vi "Replace.vi"(6 "Variant in":variant caption="变体输入", 7 "Shift Pressed?":bool caption="按下Shift？", 8 "error in (no error)":errorcluster caption="错误输入（无错误）", 10 "QD Combo Box Ref":refnum<vi> caption="快速放置组合框引用", 11 "QD Launch VI Ref":refnum<vi> caption="快速放置启动VI引用") -> (0 "error out":errorcluster caption="错误输出", 4 "Variant out":variant caption="变体输出")   [LabVIEW 2016]
doc: "将前面板或程序框图中选定的对象替换为快速放置对话框中通过名称指定的对象。\n\n默认快捷键 - [P]"
panel:
  in  "Select a Control":string="选择控件..." caption="选择控件"
  in  "Select a VI":string="选择VI..." caption="选择VI"
  in  "Undo Name":string="替换" caption="撤消名称"
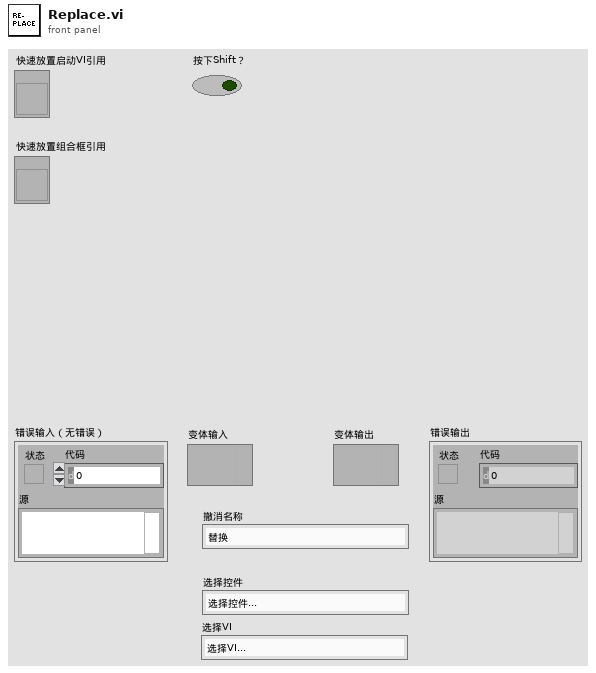
[diagram p1: front panel]
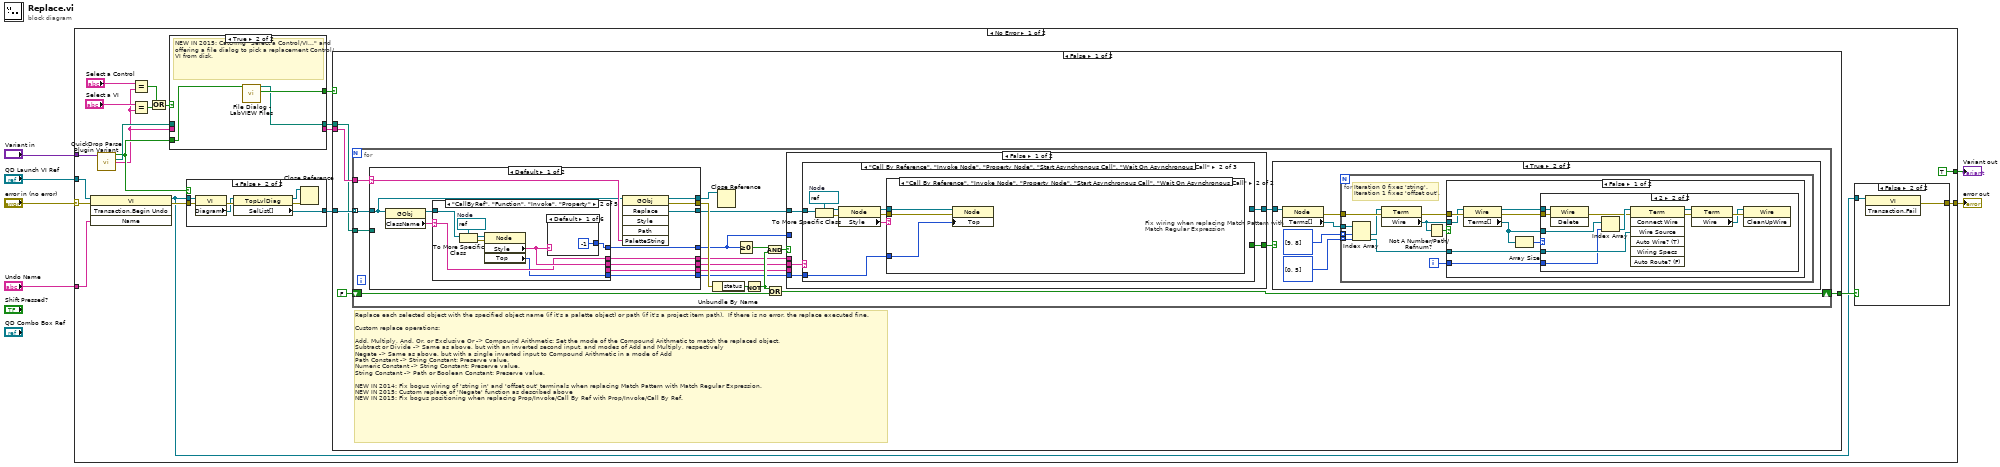
[diagram p0: block diagram]
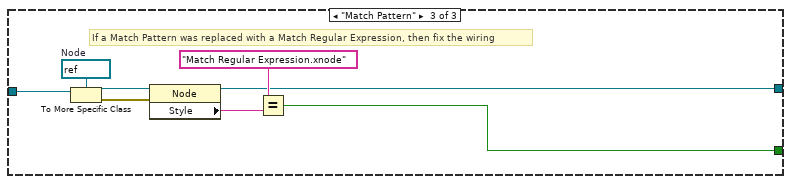
[diagram p7: hidden frame]
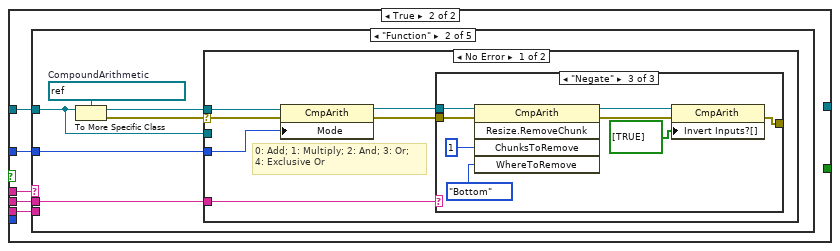
[diagram p8: hidden frame]
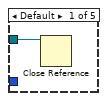
[diagram p9: hidden frame]
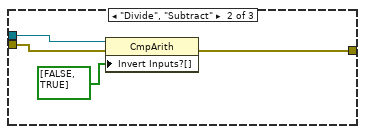
[diagram p11: hidden frame]
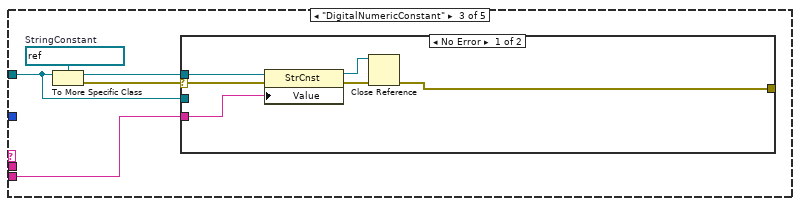
[diagram p13: hidden frame]
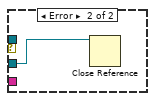
[diagram p14: hidden frame]
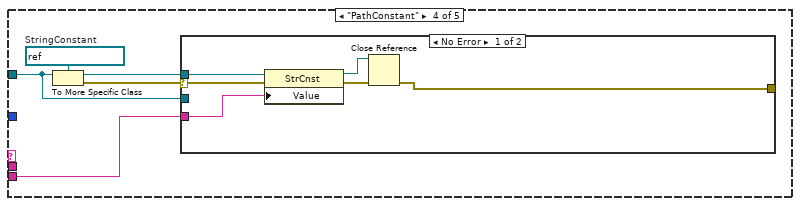
[diagram p15: hidden frame]
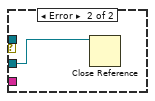
[diagram p16: hidden frame]
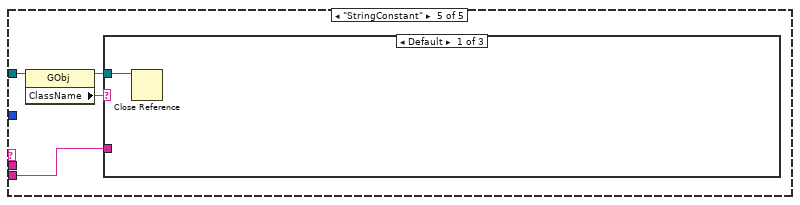
[diagram p17: hidden frame]
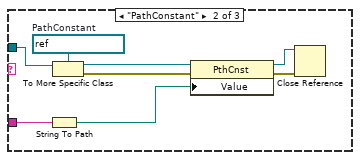
[diagram p18: hidden frame]
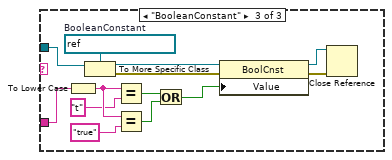
[diagram p19: hidden frame]
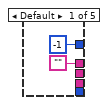
[diagram p20: hidden frame]
diagram:
  n1 = case shown="No Error" "error in (no error)" {
    selector: "error in (no error)" -> [w26 w271]
    tunnel: [w21 w271] -> w5
    tunnel: "QD Launch VI Ref" -> [w25 _]
    tunnel: "Variant in" -> [w27 _]
    tunnel: "Undo Name" -> [w24 _]
    tunnel: [TRUE _] -> w1
    frame No Error {
      n2 = invoke class="VI" method="Transaction.Begin Undo"(reference=w25, error in=w26, "Name"=w24) -> (reference out=w13:refnum<vi>, error out=w22:errorcluster)  [unwired: 1 in, 2 out]
      n3 = call <vilib>:"QuickDrop Parse Plugin Variant.vi"("QDKS Variant in"=w27) -> ("QD Launch VI Panel?"=w11:bool, "Project VI Path"=w15:path, "Palette Object Name"=w10:string)  [unwired: 12 in]
      n4 = Equal?(x="Select a Control", y=w10) -> (x = y?=w7:bool)
      n5 = Equal?(x="Select a VI", y=w10) -> (x = y?=w17:bool)
      n6 = Or(x=w7, y=w17) -> (x .or. y?=w8:bool)
      n7 = case shown="True" w8 {
        tunnel: w10 -> [w249 _]
        tunnel: w15 -> [w248 _]
        tunnel: [w249 _] -> w16
        tunnel: [w248 w251] -> w14
        tunnel: [_ w252] -> w12
        tunnel: w11 -> [_ w250]
        frame False {
        }
        frame True {
          # "NEW IN 2015: Catching \"Select a Control/VI...\" and offering a file dialog to pick a replacement Control/VI from disk."
          n8 = call <vilib>:"File Dialog - LabVIEW Files.vi"("Panel? (F)"=w250) -> ("cancelled"=w252:bool, "Path to LabVIEW File"=w251:path)  [unwired: 9 in]
        }
      }
      n9 = case shown="False" w11 {
        tunnel: w22 -> [w263 w270]
        tunnel: w13 -> [w262 w269]
        tunnel: [w257 w264] -> w19
        frame True {
          n10 = property class="VI"(reference=w262, error in=w263) -> (error out=w261:errorcluster, "Panel"=w260:refnum<vi>)  [unwired: 1 out]
          n11 = property class="Pnl"(reference=w260, error in=w261) -> (reference out=w258:refnum<vi>, error out=w259:errorcluster, "SelList[]"=w257:refnum<vi>[])
          n12 = Close Reference(reference=w258, error in (no error)=w259) -> ()  [unwired: 1 out]
        }
        frame False {
          n13 = property class="VI"(reference=w269, error in=w270) -> (error out=w268:errorcluster, "Diagram"=w267:refnum<vi>)  [unwired: 1 out]
          n14 = property class="TopLvlDiag"(reference=w267, error in=w268) -> (reference out=w265:refnum<vi>, error out=w266:errorcluster, "SelList[]"=w264:refnum<vi>[])
          n15 = Close Reference(reference=w265, error in (no error)=w266) -> ()  [unwired: 1 out]
        }
      }
      n16 = case shown="False" w12 {
        tunnel: [w31 _] -> w20
        tunnel: w19 -> [w30 _]
        tunnel: w16 -> [w29 _]
        tunnel: w14 -> [w28 _]
        frame False {
          # "Replace each selected object with the specified object name (if it's a palette object) or path (if it's a project item path).  If there is no error, the replace executed fine.\n\nCustom replace operations:\n\nAdd, Multiply, And, Or, or Exclusive Or -> Compound Arithmetic: Set the mode of the Compound Arithmetic to match the replaced object.\nSubtract or Divide -> Same as above, but with an inverted second input, and modes of Add and Multiply, respectively\nNegate -> Same as above, but with a single inverted input to Compound Arithmetic in a mode of Add\nPath Constant -> String Constant: Preserve value.\nNumeric Constant -> String Constant: Preserve value.\nString Constant -> Path or Boolean Constant: Preserve value.\n\nNEW IN 2014: Fix bogus wiring of 'string in' and 'offset out' terminals when replacing Match Pattern with Match Regular Expression.\nNEW IN 2015: Custom replace of 'Negate' function as described above\nNEW IN 2015: Fix bogus positioning when replacing Prop/Invoke/Call By Ref with Prop/Invoke/Call By Ref."
          n17 = for {
            shift-right: [w50] -> w31
            shift-left: FALSE -> [w51]
            tunnel: w30 -> [w42] mode=indexing
            tunnel: w29 -> [w49]
            tunnel: w28 -> [w48]
            n18 = case shown="Default" w49 {
              selector: w49 -> [w200 _]
              tunnel: w42 -> [w192 w247]
              tunnel: [w202 w246] -> w43
              tunnel: [w201 w245] -> w41
              tunnel: w48 -> [_ w244]
              tunnel: [w199 w243] -> w47
              tunnel: [w198 -1] -> w40
              tunnel: [w195 _] -> w38
              tunnel: [w194 _] -> w37
              tunnel: [w193 _] -> w36
              tunnel: [w191 _] -> w33
              frame Default {
                n19 = property class="GObj"(reference=w192) -> (reference out=w196:refnum<vi>, "ClassName"=w197:string)  [unwired: 1 in, 1 out]
                n20 = case shown="\"CallByRef\", \"Function\", \"Invoke\", \"Property\"" w197 {
                  selector: w197 -> [_ w206 w223 w232 w240]
                  tunnel: [-1 ("index of element") w208 0 ("index of element") 0 ("index of element") 0 ("index of element")] -> w198
                  tunnel: w196 -> [_ w209 w222 w231 w239]
                  tunnel: ["" w206 w223 w232 w240] -> w195
                  tunnel: [_ _ w219 w225 w234] -> w194
                  tunnel: [_ w207 _ _ _] -> w193
                  tunnel: [_ w205 _ _ _] -> w191
                  frame Default {
                  }
                  frame "CallByRef", "Function", "Invoke", "Property" {
                    w212 = refnum<vi> refnum  # Node
                    n21 = To More Specific Class(target class=w212, reference=w209) -> (specific class reference=w210:refnum<vi>, error out=w211:errorcluster)  [unwired: 1 in]
                    n22 = property class="Node"(reference=w210, error in=w211) -> ("Style"=w207:string, "Top"=w205:i32)  [unwired: 2 out]
                    n23 = case shown="Default" w207 {
                      tunnel: [-1 0 1 2 3 4] -> w208
                      frame Default {
                      }
                      frame "Add", "Negate", "Subtract" {
                      }
                      frame "Divide", "Multiply" {
                      }
                      frame "And" {
                      }
                      frame "Or" {
                      }
                      frame "Exclusive Or" {
                      }
                    }
                  }
                  frame "DigitalNumericConstant" {
                    w221 = refnum<vi> refnum  # DigitalNumericConstant
                    n24 = To More Specific Class(target class=w221, reference=w222) -> (specific class reference=w220:refnum<vi>)  [unwired: 1 in, 1 out]
                    n25 = property class="DigCnst"(reference=w220) -> ("NumText.Text"=w219:string)  [unwired: 1 in, 2 out]
                  }
                  frame "PathConstant" {
                    w230 = refnum<vi> refnum  # PathConstant
                    n26 = To More Specific Class(target class=w230, reference=w231) -> (specific class reference=w229:refnum<vi>)  [unwired: 1 in, 1 out]
                    n27 = property class="PthCnst"(reference=w229) -> ("Value"=w228:variant)  [unwired: 1 in, 2 out]
                    n28 = Variant To Data(type=path "", Variant=w228) -> (data=w226:path)  [unwired: 1 in, 1 out]
                    n29 = Path To String(path=w226) -> (string=w225:string)
                  }
                  frame "StringConstant" {
                    w238 = refnum<vi> refnum  # StringConstant
                    n30 = To More Specific Class(target class=w238, reference=w239) -> (specific class reference=w237:refnum<vi>)  [unwired: 1 in, 1 out]
                    n31 = property class="StrCnst"(reference=w237) -> ("Value"=w236:variant)  [unwired: 1 in, 2 out]
                    n32 = Variant To Data(type="", Variant=w236) -> (data=w234:string)  [unwired: 1 in, 1 out]
                  }
                }
                n33 = invoke class="GObj" method="Replace"(reference=w192, "PaletteString"=w200) -> (reference out=w201:refnum<vi>, error out=w199:errorcluster, "Replace"=w202:refnum<vi>)  [unwired: 4 in, 3 out]
              }
              frame "" {
                n34 = invoke class="GObj" method="Replace"(reference=w247, "Path"=w244) -> (reference out=w245:refnum<vi>, error out=w243:errorcluster, "Replace"=w246:refnum<vi>)  [unwired: 4 in, 3 out]
              }
            }
            n35 = Unbundle By Name(w47) -> ("status"=w46:bool)
            n36 = Close Reference(reference=w41) -> ()  [unwired: 1 in, 1 out]
            n37 = Greater Or Equal To 0?(x=w40) -> (x >= 0?=w39:bool)
            n38 = Not(x=w46) -> (.not. x?=w45:bool)
            n39 = And(x=w39, y=w45) -> (x .and. y?=w44:bool)
            n40 = Or(x=w45, y=w51) -> (x .or. y?=w50:bool)
            n41 = case shown="False" w44 {
              tunnel: w43 -> [w90 w114]
              tunnel: w40 -> [_ w113]
              tunnel: w38 -> [_ w112]
              tunnel: w37 -> [_ w111]
              tunnel: w36 -> [w87 w110]
              tunnel: [w88 _] -> w35
              tunnel: [w89 _] -> w34
              tunnel: w33 -> [w86 _]
              frame False {
                n42 = case shown="\"Call By Reference\", \"Invoke Node\", \"Property Node\", \"Start Asynchronous Call\", \"Wait On Asynchronous Call\"" w87 {
                  tunnel: w90 -> [_ w95 w104]
                  tunnel: [_ _ w103] -> w89
                  tunnel: [_ _ w102] -> w88
                  tunnel: w86 -> [_ w91 _]
                  frame Default {
                  }
                  frame "Call By Reference", "Invoke Node", "Property Node", "Start Asynchronous Call", "Wait On Asynchronous Call" {
                    w98 = refnum<vi> refnum  # Node
                    n43 = To More Specific Class(target class=w98, reference=w95) -> (specific class reference=w96:refnum<vi>, error out=w97:errorcluster)  [unwired: 1 in]
                    n44 = property class="Node"(reference=w96, error in=w97) -> (reference out=w93:refnum<vi>, error out=w92:errorcluster, "Style"=w94:string)
                    n45 = case shown="\"Call By Reference\", \"Invoke Node\", \"Property Node\", \"Start Asynchronous Call\", \"Wait On Asynchronous Call\"" w94 {
                      tunnel: w93 -> [_ w101]
                      tunnel: w92 -> [_ w100]
                      tunnel: w91 -> [_ w99]
                      frame "False", Default {
                      }
                      frame "Call By Reference", "Invoke Node", "Property Node", "Start Asynchronous Call", "Wait On Asynchronous Call" {
                        n46 = property class="Node"(reference=w101, error in=w100, "Top"=w99) -> ()  [unwired: 2 out]
                      }
                    }
                  }
                  frame "Match Pattern" {
                    w109 = refnum<vi> refnum  # Node
                    # "If a Match Pattern was replaced with a Match Regular Expression, then fix the wiring"
                    n47 = To More Specific Class(target class=w109, reference=w104) -> (specific class reference=w107:refnum<vi>, error out=w108:errorcluster)  [unwired: 1 in]
                    n48 = property class="Node"(reference=w107, error in=w108) -> (reference out=w103:refnum<vi>, "Style"=w106:string)  [unwired: 1 out]
                    n49 = Equal?(x="Match Regular Expression.xnode", y=w106) -> (x = y?=w102:bool)
                  }
                }
              }
              frame True {
                n50 = case shown="\"Function\"" w112 {
                  tunnel: w114 -> [w115 w118 w142 w154 w168]
                  tunnel: w113 -> [_ w117 _ _ _]
                  tunnel: w111 -> [_ _ w141 w153 w165]
                  tunnel: w110 -> [_ w116 _ _ _]
                  frame Default {
                    n51 = Close Reference(reference=w115) -> ()  [unwired: 1 in, 1 out]
                  }
                  frame "Function" {
                    w121 = refnum<vi> refnum  # CompoundArithmetic
                    n52 = To More Specific Class(target class=w121, reference=w118) -> (specific class reference=w119:refnum<vi>, error out=w120:errorcluster)  [unwired: 1 in]
                    n53 = case shown="No Error" w120 {
                      selector: w120 -> [w126 _]
                      tunnel: w119 -> [w127 _]
                      tunnel: w118 -> [_ _]
                      tunnel: w117 -> [w125 _]
                      tunnel: w116 -> [w124 _]
                      frame No Error {
                        # "0: Add; 1: Multiply; 2: And; 3: Or;\n4: Exclusive Or"
                        n54 = property class="CmpArith"(reference=w127, error in=w126, "Mode"=w125) -> (reference out=w123:refnum<vi>, error out=w122:errorcluster)
                        n55 = case shown="\"Negate\"" w124 {
                          tunnel: w123 -> [_ w132 w139]
                          tunnel: w122 -> [w128 w131 w140]
                          tunnel: [w128 w129 w136] -> _
                          frame Default {
                          }
                          frame "Divide", "Subtract" {
                            n56 = property class="CmpArith"(reference=w132, error in=w131, "Invert Inputs?[]"=bool[] [FALSE, TRUE]) -> (error out=w129:errorcluster)  [unwired: 1 out]
                          }
                          frame "Negate" {
                            n57 = invoke class="CmpArith" method="Resize.RemoveChunk"(reference=w139, error in=w140, "ChunksToRemove"=u8 1 ("Chunks To Remove"), "WhereToRemove"=enum8{"Bottom", "Top"}."Bottom" ("Where To Remove")) -> (reference out=w137:refnum<vi>, error out=w138:errorcluster)  [unwired: 1 in, 3 out]
                            n58 = property class="CmpArith"(reference=w137, error in=w138, "Invert Inputs?[]"=bool[] [TRUE]) -> (error out=w136:errorcluster)  [unwired: 1 out]
                          }
                        }
                      }
                      frame Error {
                      }
                    }
                  }
                  frame "DigitalNumericConstant" {
                    w145 = refnum<vi> refnum  # StringConstant
                    n59 = To More Specific Class(target class=w145, reference=w142) -> (specific class reference=w143:refnum<vi>, error out=w144:errorcluster)  [unwired: 1 in]
                    n60 = case shown="No Error" w144 {
                      selector: w144 -> [w150 _]
                      tunnel: w143 -> [w151 _]
                      tunnel: w142 -> [_ w152]
                      tunnel: w141 -> [w147 _]
                      tunnel: [w146 _] -> _
                      frame No Error {
                        n61 = property class="StrCnst"(reference=w151, error in=w150, "Value"=w147) -> (reference out=w148:refnum<vi>, error out=w149:errorcluster)
                        n62 = Close Reference(reference=w148, error in (no error)=w149) -> (error out=w146:errorcluster)
                      }
                      frame Error {
                        n63 = Close Reference(reference=w152) -> ()  [unwired: 1 in, 1 out]
                      }
                    }
                  }
                  frame "PathConstant" {
                    w157 = refnum<vi> refnum  # StringConstant
                    n64 = To More Specific Class(target class=w157, reference=w154) -> (specific class reference=w155:refnum<vi>, error out=w156:errorcluster)  [unwired: 1 in]
                    n65 = case shown="No Error" w156 {
                      selector: w156 -> [w162 _]
                      tunnel: w155 -> [w163 _]
                      tunnel: w154 -> [_ w164]
                      tunnel: w153 -> [w159 _]
                      tunnel: [w158 _] -> _
                      frame No Error {
                        n66 = property class="StrCnst"(reference=w163, error in=w162, "Value"=w159) -> (reference out=w160:refnum<vi>, error out=w161:errorcluster)
                        n67 = Close Reference(reference=w160, error in (no error)=w161) -> (error out=w158:errorcluster)
                      }
                      frame Error {
                        n68 = Close Reference(reference=w164) -> ()  [unwired: 1 in, 1 out]
                      }
                    }
                  }
                  frame "StringConstant" {
                    n69 = property class="GObj"(reference=w168) -> (reference out=w166:refnum<vi>, "ClassName"=w167:string)  [unwired: 1 in, 1 out]
                    n70 = case shown="Default" w167 {
                      tunnel: w166 -> [w169 w177 w190]
                      tunnel: w165 -> [_ w171 w184]
                      frame Default {
                        n71 = Close Reference(reference=w169) -> ()  [unwired: 1 in, 1 out]
                      }
                      frame "PathConstant" {
                        w176 = refnum<vi> refnum  # PathConstant
                        n72 = String To Path(string=w171) -> (path=w170:path)
                        n73 = To More Specific Class(target class=w176, reference=w177) -> (specific class reference=w174:refnum<vi>, error out=w175:errorcluster)  [unwired: 1 in]
                        n74 = property class="PthCnst"(reference=w174, error in=w175, "Value"=w170) -> (reference out=w172:refnum<vi>, error out=w173:errorcluster)
                        n75 = Close Reference(reference=w172, error in (no error)=w173) -> ()  [unwired: 1 out]
                      }
                      frame "BooleanConstant" {
                        w189 = refnum<vi> refnum  # BooleanConstant
                        n76 = To Lower Case(string=w184) -> (all lower case string=w183:string)
                        n77 = To More Specific Class(target class=w189, reference=w190) -> (specific class reference=w187:refnum<vi>, error out=w188:errorcluster)  [unwired: 1 in]
                        n78 = Equal?(x=w183, y="t") -> (x = y?=w182:bool)
                        n79 = Equal?(x=w183, y="true") -> (x = y?=w181:bool)
                        n80 = Or(x=w182, y=w181) -> (x .or. y?=w180:bool)
                        n81 = property class="BoolCnst"(reference=w187, error in=w188, "Value"=w180) -> (reference out=w185:refnum<vi>, error out=w186:errorcluster)
                        n82 = Close Reference(reference=w185, error in (no error)=w186) -> ()  [unwired: 1 out]
                      }
                    }
                  }
                }
              }
            }
            n83 = case "Fix wiring when replacing Match Pattern with Match Regular Expression" shown="True" w35 {
              tunnel: w34 -> [_ w56]
              frame False {
              }
              frame True {
                n84 = property class="Node"(reference=w56) -> (error out=w54:errorcluster, "Terms[]"=w55:refnum<vi>[])  [unwired: 1 in, 1 out]
                n85 = for {
                  tunnel: w55 -> [w66]
                  tunnel: i32[] [9, 8] -> [w65] mode=indexing
                  tunnel: i32[] [0, 5] -> [w64] mode=indexing
                  tunnel: w54 -> [w63]
                  i -> [w57]
                  # "Iteration 0 fixes 'string'.\nIteration 1 fixes 'offset out'."
                  n86 = Index Array(array=w66, index #1=w65, index #2=w64) -> (element #1=w62:refnum<vi>, element #2=w58:refnum<vi>)
                  n87 = property class="Term"(reference=w62, error in=w63) -> (error out=w60:errorcluster, "Wire"=w59:refnum<vi>)  [unwired: 1 out]
                  n88 = Not A Number/Path/Refnum?(number/path/refnum=w59) -> (NaN/Path/Refnum?=w61:bool)
                  n89 = case shown="False" w61 {
                    tunnel: w60 -> [w74 _]
                    tunnel: w59 -> [w73 _]
                    tunnel: w58 -> [w70 _]
                    tunnel: w57 -> [w67 _]
                    frame False {
                      n90 = property class="Wire"(reference=w73, error in=w74) -> (reference out=w71:refnum<vi>, error out=w72:errorcluster, "Terms[]"=w69:refnum<vi>[])
                      n91 = Array Size(array=w69) -> (size(s)=w68:i32)
                      n92 = case shown="2" w68 {
                        tunnel: w72 -> [_ w85]
                        tunnel: w71 -> [_ w76]
                        tunnel: w70 -> [_ w84]
                        tunnel: w69 -> [_ w78]
                        tunnel: w67 -> [_ w75]
                        frame Default {
                          # "Don't try to rewire with wires with multiple sinks. We would have to delete the entire wire and rewire all the sinks. This may screw up the wiring appearance in the original diagram. This check would not be necessary if the \"Delete Joint\" method of the Wire class is ever implemented."
                        }
                        frame 2 {
                          n93 = invoke class="Wire" method="Delete"(reference=w76, error in=w85) -> (error out=w77:errorcluster)  [unwired: 1 in, 2 out]
                          n94 = Index Array(array=w78, index=w75) -> (element=w79:refnum<vi>)
                          n95 = invoke class="Term" method="Connect Wire"(reference=w79, error in=w77, "Wire Source"=w84) -> (reference out=w82:refnum<vi>, error out=w83:errorcluster)  [unwired: 4 in, 5 out]
                          n96 = property class="Term"(reference=w82, error in=w83) -> (error out=w81:errorcluster, "Wire"=w80:refnum<vi>)  [unwired: 1 out]
                          n97 = invoke class="Wire" method="CleanUpWire"(reference=w80, error in=w81) -> ()  [unwired: 1 in, 3 out]
                        }
                      }
                    }
                    frame True {
                      # "Don't do anything if the terminal is unwired."
                    }
                  }
                }
              }
            }
          }
        }
        frame True {
        }
      }
      n98 = case shown="False" w20 {
        tunnel: w13 -> [w253 w255]
        tunnel: [w254 w256] -> w21
        frame True {
          n99 = invoke class="VI" method="Transaction.End Undo"(reference=w253) -> (error out=w254:errorcluster)  [unwired: 2 in, 2 out]
        }
        frame False {
          n100 = invoke class="VI" method="Transaction.Fail"(reference=w255) -> (error out=w256:errorcluster)  [unwired: 2 in, 2 out]
        }
      }
    }
    frame Error {
    }
  }
  "error out" <- w5
  "Variant out" <- w1
